vi "Input.vi"(9 "Module Info In":T1, 11 "Engine Tags In":T3) -> (1 "Module Info Out":T1, 3 "Engine Tags Out":T3)   [LabVIEW 2013, in "synchronous engine runtime.lvclass"]
uses:
  synchronous engine runtime.lvclass
  <vilib>/NI/Tag Bus/table/data table.ctl
  Module Execution Info.ctl
  <vilib>/NI/Tag Bus Module Framework/runtime/TBM module execution interface.lvclass
  Data Table with Transfer Spec.ctl
  <vilib>/NI/Tag Bus/table/transfer specification.ctl
  <vilib>/NI/Tag Bus/tag/Data Type.ctl
  <vilib>/NI/Tag Bus/table/data table.lvlib
  <vilib>/NI/Tag Bus/tag/tag descriptor.lvclass
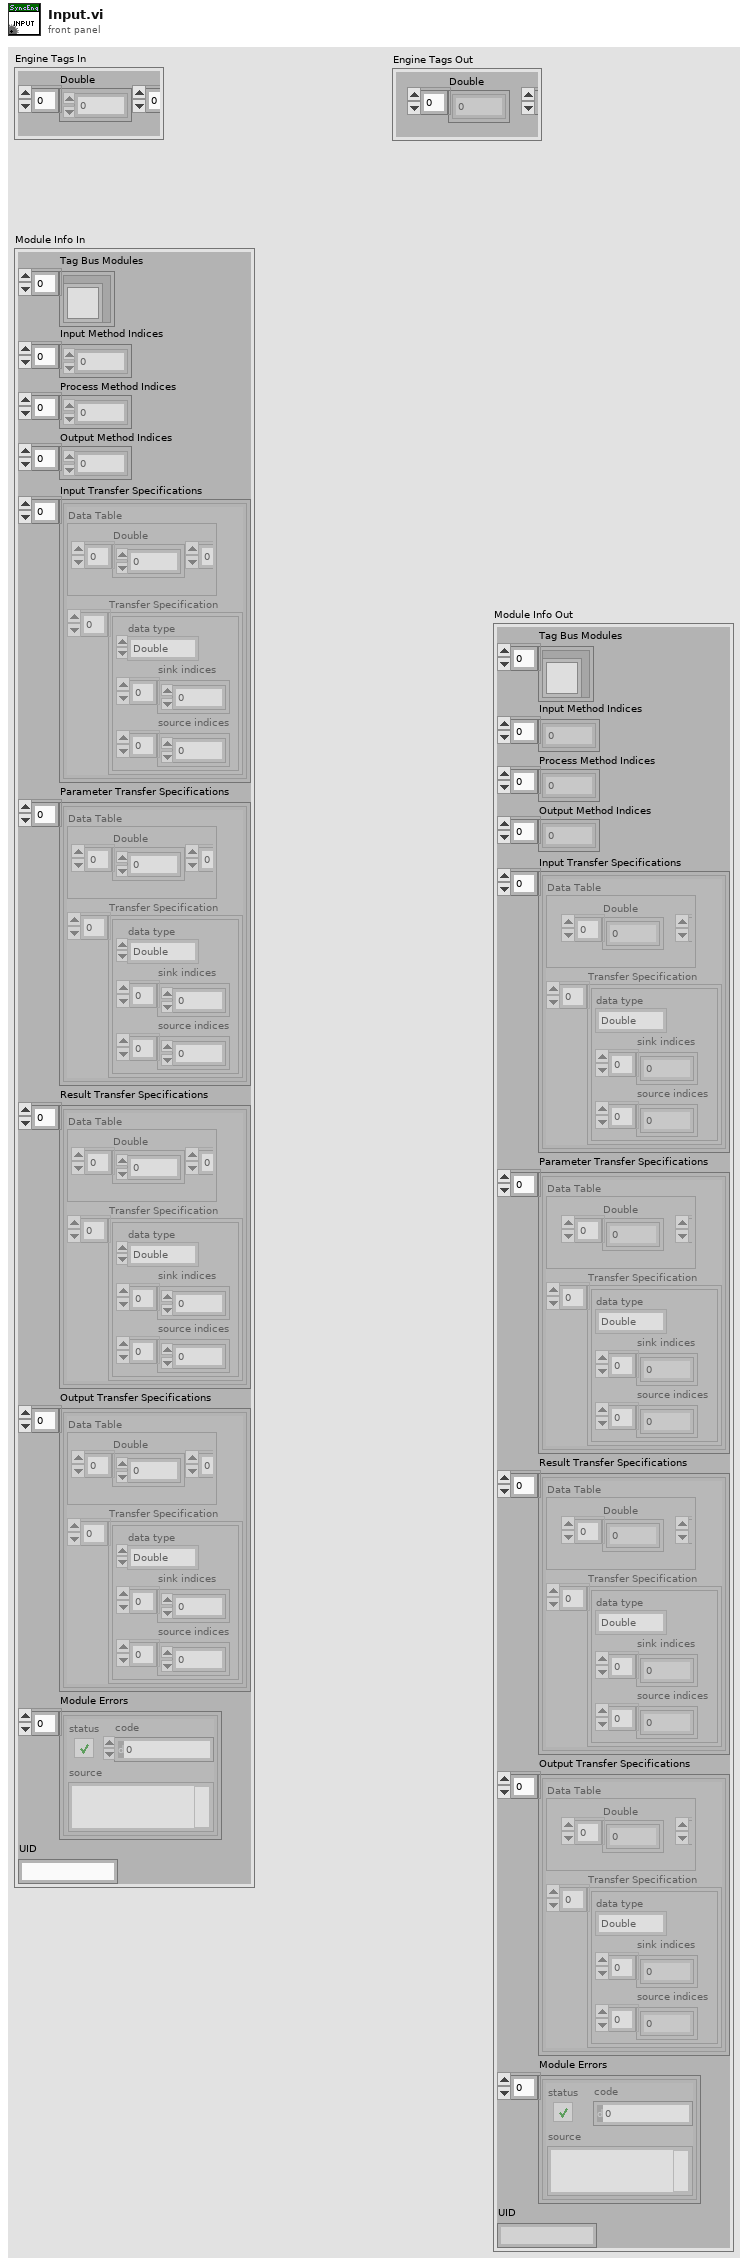
[diagram p1: front panel]
types:
  T1 = typedef "synchronous engine runtime.lvclass/Module Execution Info.ctl" = cluster{"Tag Bus Modules":refnum<class "TBM module execution interface.lvclass">[], "Input Method Indices":i32[], "Process Method Indices":i32[], "Output Method Indices":i32[], "Input Transfer Specifications":T2[], "Parameter Transfer Specifications":T2[], "Result Transfer Specifications":T2[], "Output Transfer Specifications":T2[], "Module Errors":errorcluster[], "UID":string}
  T2 = typedef "synchronous engine runtime.lvclass/Data Table with Transfer Spec.ctl" = cluster{"Data Table":T3, "Transfer Specification":T4[]}
  T3 = typedef "tag bus.lvlib/data table.lvlib/data table.ctl" = cluster{"Double":dbl[], "Single":sgl[], "I64":i64[], "I32":i32[], "I16":i16[], "I8":i8[], "U64":u64[], "U32":u32[], "U16":u16[], "U8":u8[], "Boolean":bool[], "String":string[], "Array of Double":cluster{"DBL Array":dbl[]}[], "Array of Single":cluster{"SGL Array":sgl[]}[], "Array of I64":cluster{"I64 Array":i64[]}[], "Array of I32":cluster{"I32 Array":i32[]}[], "Array of I16":cluster{"I16 Array":i16[]}[], "Array of I8":cluster{"I8 Array":i8[]}[], "Array of U64":cluster{"U64 Array":u64[]}[], "Array of U32":cluster{"U32 Array":u32[]}[], "Array of U16":cluster{"U16 Array":u16[]}[], "Array of U8":cluster{"U8 Array":u8[]}[], "Array of Boolean":cluster{"Boolean Array":bool[]}[], "Array of String":cluster{"String Array":string[]}[]}
  T4 = typedef "tag bus.lvlib/data table.lvlib/transfer specification.ctl" = cluster{"data type":T5, "sink indices":i32[], "source indices":i32[]}
  T5 = typedef "tag bus.lvlib/tag descriptor.lvclass/Data Type.ctl" = enum16{"Double", "Single", "I64", "I32", "I16", "I8", "U64", "U32", "U16", "U8", "Boolean", "String", "Array of Double", "Array of Single", "Array of I64", "Array of I32", "Array of I16", "Array of I8", "Array of U64", "Array of U32", "Array of U16", "Array of U8", "Array of Boolean", "Array of String"}
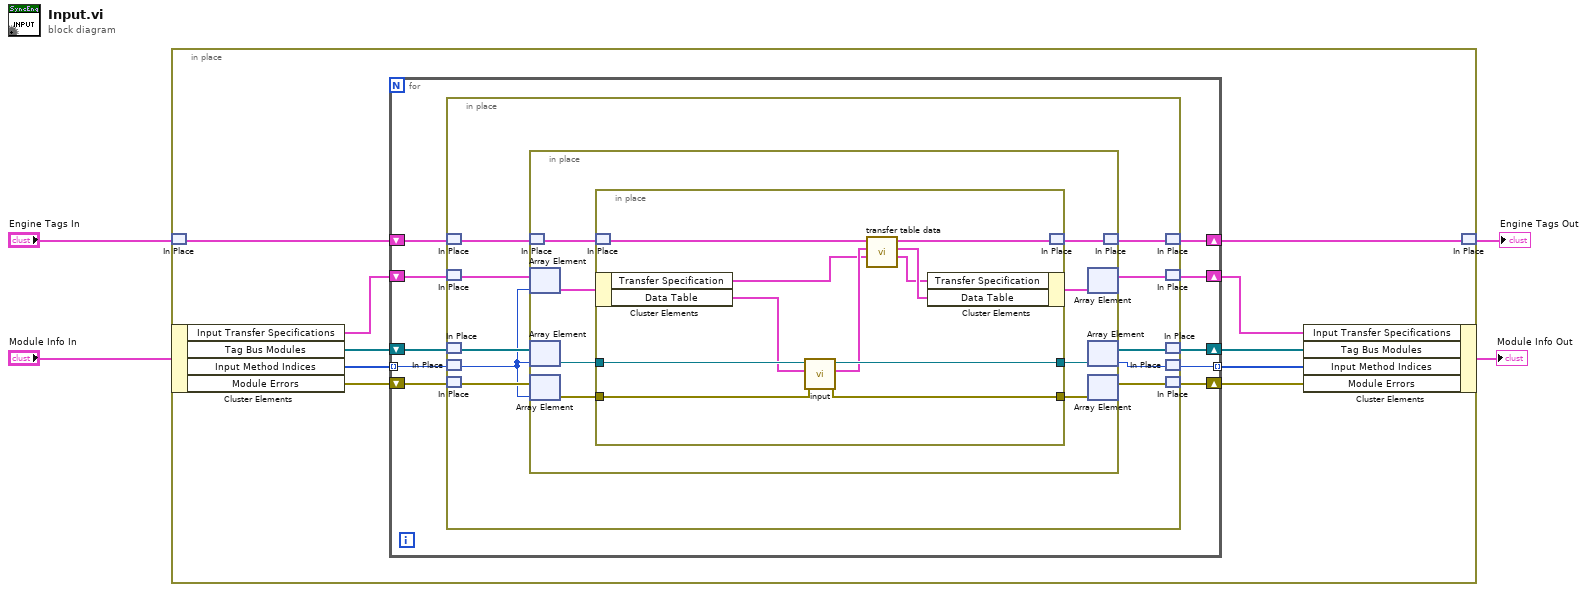
[diagram p0: block diagram]
diagram:
  n1 = in-place {
    n2 = in-place-match #1("Engine Tags In") -> (w13:T3)
    n3 = in-place-cluster #2("Module Info In") -> ("Input Transfer Specifications"=w11:T2[], "Tag Bus Modules"=w8:refnum<class "TBM module execution interface.lvclass">[], "Input Method Indices"=w14:i32[], "Module Errors"=w10:errorcluster[])
    n4 = for {
      shift-right: [w19] -> w7
      shift-left: w8 -> [w20]
      tunnel: w14 -> [w16] mode=indexing
      shift-right: [w23] -> w12
      shift-left: w13 -> [w24]
      shift-right: [w21] -> w9
      shift-left: w11 -> [w22]
      shift-right: [w17] -> w6
      shift-left: w10 -> [w18]
      tunnel: [w15] -> w5 mode=indexing
      n5 = in-place {
        n6 = in-place-match #3(w24) -> (w34:T3)
        n7 = in-place-match #4(w22) -> (w32:T2[])
        n8 = in-place-match #5(w20) -> (w30:refnum<class "TBM module execution interface.lvclass">[])
        n9 = in-place-match #6(w16) -> (w26:i32)
        n10 = in-place-match #7(w18) -> (w28:errorcluster[])
        n11 = in-place {
          n12 = in-place-match #8(w34) -> (w38:T3)
          n13 = in-place-array #9(w32, w26) -> (w36:T2)
          n14 = in-place-array #10(w30, w26) -> (w42:refnum<class "TBM module execution interface.lvclass">)
          n15 = in-place-array #11(w28, w26) -> (w41:errorcluster)
          n16 = in-place {
            in-place-border: w42 -> [w53]
            in-place-border: w41 -> [w52]
            in-place-border: [w51] -> w40
            in-place-border: [w43] -> w39
            n17 = in-place-match #12(w38) -> (w49:T3)
            n18 = in-place-cluster #13(w36) -> ("Transfer Specification"=w45:T4[], "Data Table"=w47:T3)
            n19 = call-dynamic "input.vi"("error in"=w52, "input allocation"=w47, "module in"=w53) -> ("error out"=w43:errorcluster, "input data"=w50:T3, "module out"=w51:refnum<class "TBM module execution interface.lvclass">)  [unwired: 6 in]
            n20 = call <vilib>:"transfer table data.vi"("transfer specification in"=w45, "data table source in"=w50, "data table sink in"=w49) -> ("transfer specification out"=w44:T4[], "data table source out"=w46:T3, "data table sink out"=w48:T3)  [unwired: 6 in]
            n21 = in-place-cluster #13("Transfer Specification"=w44, "Data Table"=w46) -> (w35:T2)
            n22 = in-place-match #12(w48) -> (w37:T3)
          }
          n23 = in-place-array #9(w35) -> (w31:T2[])  [unwired: 1 out]
          n24 = in-place-array #10(w40) -> (w29:refnum<class "TBM module execution interface.lvclass">[], w25:i32)
          n25 = in-place-array #11(w39) -> (w27:errorcluster[])  [unwired: 1 out]
          n26 = in-place-match #8(w37) -> (w33:T3)
        }
        n27 = in-place-match #3(w33) -> (w23:T3)
        n28 = in-place-match #4(w31) -> (w21:T2[])
        n29 = in-place-match #5(w29) -> (w19:refnum<class "TBM module execution interface.lvclass">[])
        n30 = in-place-match #6(w25) -> (w15:i32)
        n31 = in-place-match #7(w27) -> (w17:errorcluster[])
      }
    }
    n32 = in-place-cluster #2("Input Transfer Specifications"=w9, "Tag Bus Modules"=w7, "Input Method Indices"=w5, "Module Errors"=w6) -> (→"Module Info Out":T1)
    n33 = in-place-match #1(w12) -> (→"Engine Tags Out":T3)
  }
